vi "Add Registered Process.vi"(4 "Sync Notifier":refnum<notifier>, 6 "Process Runs (T)":bool=TRUE, 8 "error in (no error)":errorcluster, 9 "Process Name (Optional)":string, 10 "Process VI (Static VI Ref)":refnum<vi>, 11 "SMO":refnum<class "SMO.lvclass">) -> (0 "error out":errorcluster, 3 "SMO out":refnum<class "SMO.lvclass">)   [LabVIEW 2013, in "SMO.lvclass"]
doc: "---------------------------------------------------------------\nCopyright © 2014 JKI All rights reserved.\nAuthor: Philippe Guerit <philippe.guerit@jki.net>\nThis library is provided \"AS IS\" , WITHOUT WARRANTIES OR \nCONDITIONS OF ANY KIND, either express or implied.\nJKI. -- jki.net"
uses:
  SMO.lvclass
  SMO.lvclass/SMO.ctl
panel:
  # "For instructions on how to use the JKI State Machine Objects, examples and video tutorials, visit:\nhttp://jki.net/state-machine-objects/\n\nJKI State Machine Objects™\nhttp://jki.net/state-machine-objects/\nCopyright (C) 2005-2015, JKI <info@jki.net>\nALL RIGHTS RESERVED"
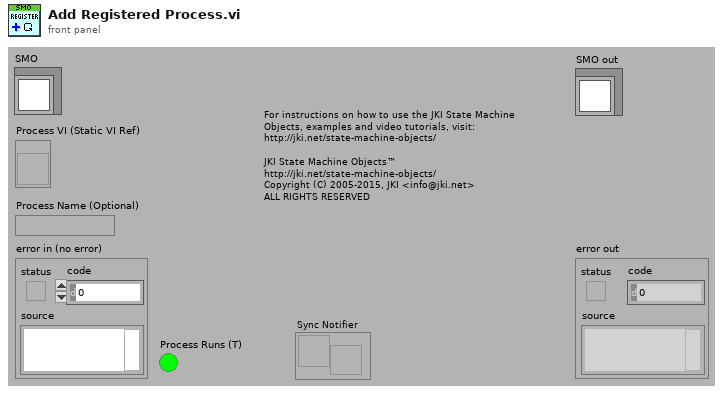
[diagram p1: front panel]
types:
  T1 = typedef "SMO.lvclass/PrivateData--Ref.ctl" = refnum<data-value>
  T2 = typedef "SMO.lvclass/PrivateData--Cluster.ctl" = cluster{"Parent Call":T3, "Registered Processes":T4[], "Sync Notifier":refnum<notifier>, "Process Error Notifier":refnum<notifier>, "Protected Events":T5, "Public Events":T6, "SMO State":T7, "[Dependencies]":T8[], "[Attributes]":refnum<class "Attribute.lvclass">[], "Launcher Close":refnum<notifier>}
  T3 = typedef "SMO.lvclass/Parent Call--Enum.ctl" = enum16{"Allows parent to run", "Does not request parent to run"}
  T4 = typedef "SMO.lvclass/RegisteredProcessData--Cluster.ctl" = cluster{"Name":string, "Static VI Ref":refnum<vi>, "Running":bool, "NotifierRef":u32}
  T5 = typedef "SMO.lvclass/Protected Events.ctl" = cluster{"StopProcesses":refnum<user-event>, "AbortProcesses":refnum<user-event>, "Config Changed":refnum<user-event>}
  T6 = typedef "SMO.lvclass/Public Events.ctl" = cluster{"Error":refnum<user-event>, "State":refnum<user-event>}
  T7 = typedef "SMO.lvclass/SMOState --Enum.ctl" = enum16{"unknown", "Created", "Started", "Stopped"}
  T8 = typedef "SMO.lvclass/SMO Dependency--Cluster.ctl" = cluster{"Dependency":refnum<class "SMO.lvclass">, "Level":string}
  T9 = cluster{"Clone Name":string, "Process VI (Static VI Ref)":refnum<vi>, "Process Runs (T)":bool, u32}
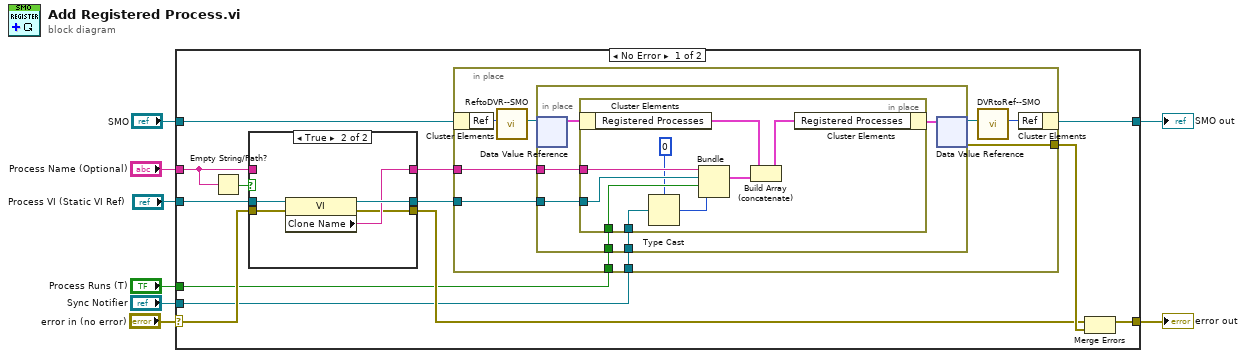
[diagram p0: block diagram]
diagram:
  n1 = case shown="No Error" "error in (no error)" {
    selector: "error in (no error)" -> [w12 w55]
    tunnel: "Process VI (Static VI Ref)" -> [w17 _]
    tunnel: [w18 w55] -> w7
    tunnel: "Process Name (Optional)" -> [w13 _]
    tunnel: [w20 w54] -> w4
    tunnel: "SMO" -> [w21 w54]
    tunnel: "Process Runs (T)" -> [w10 _]
    tunnel: "Sync Notifier" -> [w9 _]
    frame No Error {
      n2 = Empty String/Path?(string/path=w13) -> (empty?=w15:bool)
      n3 = case shown="True" w15 {
        tunnel: w17 -> [w23 w29]
        tunnel: [w23 w28] -> w16
        tunnel: [w24 w27] -> w14
        tunnel: w13 -> [w24 _]
        tunnel: w12 -> [w22 w26]
        tunnel: [w22 w25] -> w11
        frame False {
        }
        frame True {
          n4 = property class="VI"(reference=w29, error in=w26) -> (reference out=w28:refnum<vi>, error out=w25:errorcluster, "Clone Name"=w27:string)
        }
      }
      n5 = in-place {
        in-place-border: w14 -> [w38]
        in-place-border: w16 -> [w37]
        in-place-border: [w36] -> w19
        in-place-border: w10 -> [w31]
        in-place-border: w9 -> [w30]
        n6 = in-place-cluster #1(w21) -> ("Ref"=w35:u32)
        n7 = call "ReftoDVR--SMO.vi"("Ref"=w35) -> ("Ref"=w34:T1)  [unwired: 10 in]
        n8 = in-place {
          in-place-border: w38 -> [w43]
          in-place-border: w37 -> [w42]
          in-place-border: w31 -> [w40]
          in-place-border: w30 -> [w39]
          n9 = in-place-dvr #2(w34) -> (w44:T2)  [unwired: 1 out]
          n10 = in-place {
            in-place-border: w43 -> [w51]
            in-place-border: w42 -> [w50]
            in-place-border: w40 -> [w48]
            in-place-border: w39 -> [w46]
            n11 = in-place-cluster #3(w44) -> ("Registered Processes"=w53:T4[])
            n12 = Type Cast(type=u32 0, x=w46) -> (*(type *) &x=w45:u32)
            n13 = Bundle("Clone Name"=w51, "Process VI (Static VI Ref)"=w50, "Process Runs (T)"=w48, w45) -> (w49:T9)  [unwired: 1 in]
            n14 = Build Array (concatenate)(w53, w49) -> (w52:T4[])
            n15 = in-place-cluster #3("Registered Processes"=w52) -> (w41:T2)
          }
          n16 = in-place-dvr #2(w41) -> (w33:T1, w36:errorcluster)
        }
        n17 = call "DVRtoRef--SMO.vi"("Ref"=w33) -> ("Ref"=w32:u32)  [unwired: 10 in]
        n18 = in-place-cluster #1("Ref"=w32) -> (w20:refnum<class "SMO.lvclass">)
      }
      n19 = Merge Errors(w11, w19) -> (w18:errorcluster)
    }
    frame Error {
    }
  }
  "error out" <- w7
  "SMO out" <- w4
